vi "Increment Load Wheel.vi"() -> (14 "Splash Indicator Cluster out":T1)   [LabVIEW 2020]
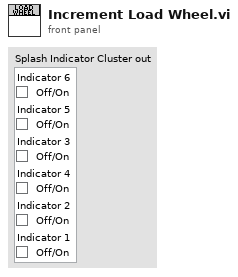
[diagram p1: front panel]
types:
  T1 = cluster{"Indicator 6":bool, "Indicator 5":bool, "Indicator 3":bool, "Indicator 4":bool, "Indicator 2":bool, "Indicator 1":bool}
  T2 = cluster{"[0]":bool, "[1]":bool, "[2]":bool, "[3]":bool, "[4]":bool, "[5]":bool, "[6]":bool, "[7]":bool, "[8]":bool}
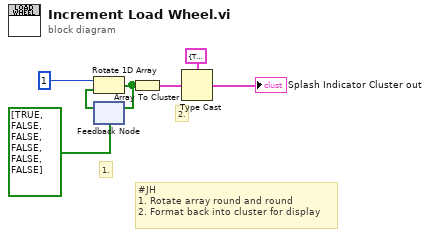
[diagram p0: block diagram]
diagram:
  # "#JH\n1. Rotate array round and round\n2. Format back into cluster for display"
  # "2."
  # "1."
  n1 = feedback #1(bool[] [TRUE, FALSE, FALSE, FALSE, FALSE, FALSE]) -> (w2:bool[])
  n2 = Rotate 1D Array(1:w2, 2:1 ("Count")) -> (0:w3:bool[])
  n3 = feedback-in #1(w3) -> ()
  n4 = Array To Cluster(array=w3) -> (cluster=w6:T2)
  n5 = Type Cast(type=T1 {"Indicator 6"=TRUE, "Indicator 5"=TRUE, "Indicator 3"=TRUE, "Indicator 4"=TRUE, "Indicator 2"=TRUE, "Indicator 1"=TRUE} ("Splash Indicator Cluster"), x=w6) -> (*(type *) &x=→"Splash Indicator Cluster out":T1)
